vi "Set All Names and Values.vi"(0 "Variant (Cluster) In":variant, 5 "Name":string, 7 "Element Names":string[](array[string]), 9 "values":variant[](array[variant]), 11 "error in":errorcluster) -> (4 "Variant (Cluster) Out":variant, 15 "error out":errorcluster)   [LabVIEW 2017, in "Advanced Variant Tools.lvlib"]
doc: "Returns an array of all of the keys and an array of their corresponding values. Elements are correlated by index, so the key at a given index corresponds to the value at the same index."
uses:
  Advanced Variant Tools.lvlib
  <vilib>/Utility/Data Type/NI_Data Type.lvlib
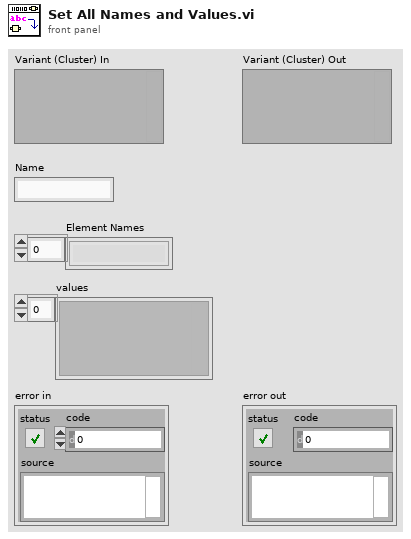
[diagram p1: front panel]
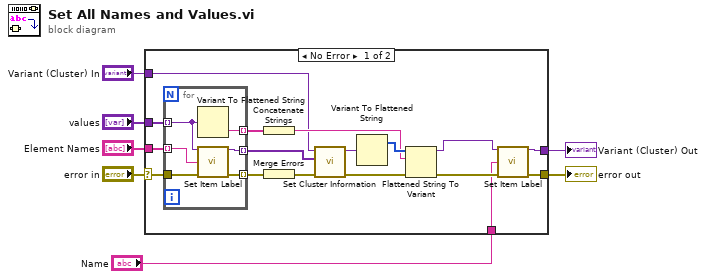
[diagram p0: block diagram]
diagram:
  n1 = case shown="No Error" "error in" {
    selector: "error in" -> [w13 w31]
    tunnel: "Variant (Cluster) In" -> [w10 w32]
    tunnel: "values" -> [w18 _]
    tunnel: [w15 w32] -> w5
    tunnel: [w14 w31] -> w3
    tunnel: "Element Names" -> [w19 _]
    tunnel: "Name" -> [w8 _]
    frame No Error {
      n2 = for {
        tunnel: w18 -> [w27] mode=indexing
        tunnel: [w30] -> w24 mode=indexing
        tunnel: w19 -> [w29] mode=indexing
        tunnel: [w28] -> w17 mode=indexing
        tunnel: w13 -> [w26]
        tunnel: [w25] -> w12 mode=indexing
        n3 = Variant To Flattened String(Variant=w27) -> (data string=w30:string)  [unwired: 1 out]
        n4 = call "Set Item Label.vi"("Variant in"=w27, "Name"=w29, "error in (no error)"=w26) -> ("Variant out"=w28:variant, "error out"=w25:errorcluster)  [unwired: 11 in]
      }
      n5 = Concatenate Strings(w24) -> (w21:string)
      n6 = Merge Errors(w12) -> (w11:errorcluster)
      n7 = call <vilib>:"Set Cluster Information.vi"("error in (no error)"=w11, "Cluster Elements"=w17, "Variant in"=w10) -> ("error out"=w20:errorcluster, "Variant out"=w23:variant)  [unwired: 7 in]
      n8 = Variant To Flattened String(Variant=w23) -> (1:w22:i16[])  [unwired: 1 out]
      n9 = Flattened String To Variant(4:w20, 6:w21, 7:w22) -> (0:w9:errorcluster, 3:w16:variant)
      n10 = call "Set Item Label.vi"("Variant in"=w16, "Name"=w8, "error in (no error)"=w9) -> ("Variant out"=w15:variant, "error out"=w14:errorcluster)  [unwired: 11 in]
    }
    frame Error {
    }
  }
  "error out" <- w3
  "Variant (Cluster) Out" <- w5
